vi "AutoNav 1.vi"   [LabVIEW 2009]
uses:
  <vilib>/NXT/Block Support/NXT_InputPort.ctl
  <vilib>/NXT/Block Support/NXT_OutputPort.ctl
  <vilib>/NXT/Dual Mode Library/Display/drawText.vi
  <vilib>/NXT/Dual Mode Library/Sensors/Sonar_cm.vi
types:
  T1 = typedef "NXT_OutputPort.ctl" = u8
  T2 = typedef "NXT_InputPort.ctl" = u8
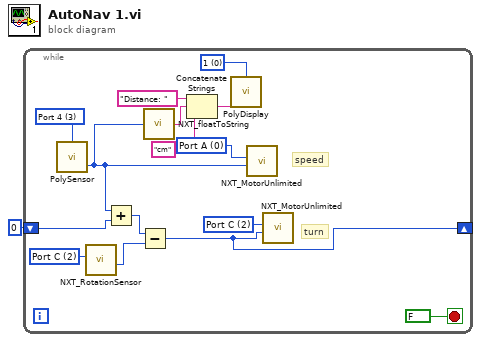
[diagram p0: block diagram]
diagram:
  n1 = while {
    shift-right: [w2] -> _
    shift-left: 0 -> [w7]
    stop <- FALSE stop-if-true
    w5 = T1 2 items=["Port A", "Port B", "Port C"] ("Output (Port A)")
    w6 = T1 2 items=["Port A", "Port B", "Port C"] ("Output (Port A)")
    w10 = T1 0 items=["Port A", "Port B", "Port C"] ("Output (Port A)")
    w11 = T2 3 items=["Port 1", "Port 2", "Port 3", "Port 4"] ("Port (Port 4)")
    w12 = i16 0 items=["1", "2", "3", "4", "5", "6", "7", "8"] ("Line")
    # "turn"
    # "speed"
    n2 = call-poly <vilib>:"PolySensor.vi"("Port (Port 4)"=w11) -> ("Distance (cm)"=w8:i16)  [unwired: 2 in, 1 out]
    n3 = call <vilib>:"NXT_RotationSensor.vi"("Output (Port A)"=w5) -> ("Degrees out"=w3:i32)  [unwired: 7 in, 3 out]
    n4 = Add(x=w8, y=w7) -> (x+y=w4:i32)
    n5 = Subtract(x=w4, y=w3) -> (x-y=w2:i32)
    n6 = call <vilib>:"NXT_floatToString.vi"("number"=w8) -> ("string"=w14:string)
    n7 = Concatenate Strings("Distance: " ("string"), w14, "cm" ("string")) -> (w15:string)
    n8 = call-poly <vilib>:"PolyDisplay.vi"("Text"=w15, "Line"=w12) -> ()  [unwired: 2 in, 1 out]
    n9 = call <vilib>:"NXT_MotorUnlimited.vi"("Power (75)"=w8, "Output (Port A)"=w10) -> ()  [unwired: 8 in, 2 out]
    n10 = call <vilib>:"NXT_MotorUnlimited.vi"("Power (75)"=w2, "Output (Port A)"=w6) -> ()  [unwired: 8 in, 2 out]
  }
